vi "Z-Scan-test-1.vi"() -> ()   [LabVIEW 2014]
doc: "André Romero - 2016\nandretec@ifsc.usp.br"
uses:
  <vilib>/Utility/file.llb/Write To Spreadsheet File (DBL).vi
  <vilib>/Analysis/NI_AALBase.lvlib
panel:
  out "Waveform Chart 2":u32(graph)
  out "x-y":u32
  out "mean 2":dbl format="%0.2f"
  out "Waveform Chart":u32(graph)
  out "tempo":u32
  out "points":i32=1
  out "appended array":dbl[](array[numeric])
  out "variance":dbl format="%0.4f"
  out "standard deviation":dbl format="%0.4f"
  out "mean":dbl format="%0.4f"
  in  "Save ?":bool
  in  "delay between points (ms)":u32=100
  out "Waveform Graph 2":dbl[](graph)=[0.9929619826026088, 0.9923746873025917, 0.9818508984469507, 0.983827466273251, 0.9990107623733235, 1.0395239819940292, 0.9706500523861651, 1.06794722078419, 0.986424747001235, 1.0112744316316724, 0.9942522731444444, 1.001838469740766, 1.0029946225195683, 1.0126120902171765, 1.0021644811870658, 1.0061116820401748, 0.9972105448102168, 1.0068911643301743, 1.0052132138264187, 0.9992750904172452, 1.048311614015414, 0.9926080305613119, 1.0111948048086972, 0.9905398114026907, 1.0116783915731316, 0.98387502636871, 1.0107154218811778, 0.9941931066061604, 0.9875775120102475, 0.9829757035289887, 1.0188092280445085, 1.0111453402362722, 0.9875075292482545, 0.995337740298579, 1.0079138648082209, 1.0254835549800694, 0.9939970887218519, 0.9842725457434127, 0.9855748100955501, 0.9966738309822512, 1.0098279420600873, 0.9948048737150966, 1.0135979927834378, 0.964293348097744, 1.0004442713410568, 1.0081850647456483, 1.0302507900473072, 1.0228923303488178, 0.9667484984963655, 0.9865714477739775, 1.0364133365991077, 0.9977213956061421, 0.9832428050829438, 1.0383334543535299, 1.0096732459951854, 0.9825962938516749, 1.0183344805260317, 1.0177353873122412, 1.0225410223146796, 0.9860754307269641, 1.030312013840959, 1.0285466334678401, 1.0597004685457643, 0.9964393152435648, 1.0127420032997732, 1.0111564309410899, 0.9911153373064908, 0.9829525872811106, 0.9871642314547671, 1.0194200583287394, 1.00388773598447, 0.9746341672739159, 0.9904278906168584, 1.0033900330518635, 0.9936252883479672, 0.9845205151436855, 0.9945678585238711, 1.0016647654820403, 0.9879898688451537, 0.9863984551003344, 1.0110167839368691, 0.9752355124150663, 1.0344780794239226, 1.0122843072036265, 1.01049678196296, 0.970736922329293, 1.0241881965977657, 1.0115188722181554, 1.0293585291923657, 0.9982310438764077, 1.0051149836556408, 1.017911251728115, 0.9594139388753959, 1.0078413224573917, 1.003688804255993, 1.006221484876327, 0.9967339615841198, 1.0042760036472898, 0.9537852705680492, 1.0212543549523825, 1.0183418109287485, 0.9834384603549127, 0.9725833860677029, 0.9993225762516945, 1.002606361854476, 0.9876410897688062, 1.0036466615678723, 1.0019409165776714, 0.9963709181949384, 0.9968424660158376, 0.9935766114990483, 1.0116577111029135, 0.9882456586285582, 1.0072538601971548, 1.0120599790471025, 0.9770225341272584, 1.0173265485746734, 0.9723656657261552, 1.0043411013798933, 0.972400846287812, 0.9965743699288137, 1.0115957985488486, 1.0092600598782004, 1.028617902659787, 0.9756263120391087, 1.0251995340244466, 0.9981801685348355, 1.0172999638370765, 1.0056541703390969, 0.995990126879641, 0.9963655622831015, 1.032430445611457, 1.001431336754485, 1.0006099730723665, 1.0041724165772414, 1.0053778599068968, 0.991135402560612, 0.9998817432648112, 0.9912809462492138, 1.0035465593288295, 0.9882437595283899, 0.9782107765089285, 1.0228518124206731, 1.0087558934341563, 1.0241891638206257, 1.0193787553010976, 0.9921167807164234, 0.9927502420161048, 1.0107346398658508, 1.0188837238645847, 1.0221594671883125, 0.9965942993860635, 0.9842932321001923, 0.981847030230603, 0.9936136652990707, 0.9870447044168618, 0.9978949690731117, 0.9869918626920519, 0.9797386003847882, 1.0008386985082103, 1.0330280927007673, 1.004241674125628, 0.9909683650164001, 1.02695629802514, 1.0033708015406961, 1.0108056398846754, 0.9945908054831527, 1.0155686303054825, 0.985836754279153, 1.0122873083447073, 0.9813554692374822, 1.0073229755773239, 1.0020783249839669, 1.0023809695174208, 1.0021245575406161, 1.0074700445823073, 0.9899219659902431, 0.9881872351711627, 1.0049950341400478, 1.0046843040273437, 1.0201054172795425, 0.9937380855148645, 1.0021211500967366, 1.0088570028712045, 1.0044231329331996, 0.9984501684286005, 1.0013270763238702, 0.9774971335854716, 0.9866658163334106, 1.000980775430664, 0.9908481010755628, 1.0002528700293596, 0.9857656778619052, 0.9997826772620825, 1.0343649620339501, 1.0073234584006823, 0.9805240664825804, 1.0029654601008016, 0.9686768780166081, 1.0160258125494137, 1.0082079553664105, 0.9901357158841061, 0.994748065638555, 1.0052403943152382, 0.9871031757851597, 1.0214066887952424, 0.9704901116769896, 0.9950660968868316, 1.0019640529928464, 0.9936374248988875, 1.003497863963157, 1.0093061063561608, 0.9911483093985394, 0.997450965146168, 0.9966121176455948, 0.9993526179830612, 1.0053031425218377, 0.9913746748359868, 1.0026744008784367, 1.0025305796566382, 0.9931120665299722, 0.9864936832201258, 0.9828125296228193, 1.0154017305245813, 0.999977292098376, 1.003396060860759, 1.0090206669165798, 1.0124763635969498, 1.0105591289236533, 1.0084645494960998, 0.9855441101537715, 1.0017739263357615, 1.0065720022143287, 0.9922343777252469, 0.9981592542558017, 1.0001288888719242, 1.0039210730337789, 1.012377141773532, 1.0047424479160145, 1.0014599375745836, 1.013669723894066, 1.0050191875283112, 0.9938872072614322, 1.011570859686594, 0.996138314975225, 0.9939848274478382, 1.0065053877719619, 0.9944330961628688, 0.9791961444806913, 0.9999374454812969, 0.9975934276752868, 0.9944102204807054, 0.989392831994615, 1.0115392036215836, 1.0031898996148303, 1.0146271680824552, 0.9943257833943299, 0.9988752320358599, 1.0058922758561464, 1.006497779872354, 0.9930252211908878, 1.0235100479739772, 0.9933965078745319, 0.995734537346277, 0.9921857029695909, 0.997394921680454, 1.00664676734835, 1.0018598311217508, 0.999330072011583, 0.9988076745749431, 1.0106882210145283, 0.9964673682162559, 0.9977625424375128, 0.9969296445631848, 1.0097354699541692, 0.9908315377852488, 1.001406845754614, 0.9957275654561938, 0.9999071939760551, 1.0133978457034993, 1.0005501801740915, 0.9728144753536448, 0.9788149064050354, 0.9963338202361954, 0.9901746458167859, 1.0148500134459466, 1.0007813474773088, 1.0001239602007925, 1.0003956980130249, 0.9897066956415941, 1.0152655774500954, 1.006420164781569, 0.9987813936052027, 0.997929586836126, 1.0047079456911374, 0.9987477059026443, 0.9930327363838042, 0.997335295316322, 1.0006172967849036, 0.9833077793511378, 1.0085601133813822, 0.9943971410893149, 0.994239981170442, 1.0012084094477036, 0.9970289367786878, 0.9917988514890875, 1.000045439682172, 1.0047485655661257, 1.0030878243674637, 1.0023693825498734, 0.9823961549994707, 1.0089568692112538, 1.0128225400030877, 0.993059303619402, 1.0000477118317317, 1.008386816093551, 1.0061752524742424, 1.0012782594079208, 1.0088193880168852, 0.9998113759745942, 0.9916808751924095, 0.9947764469785467, 1.0000147588767094, 1.004168257302679, 1.0049594024199107, 0.9976032955590068, 0.9950024479190206, 1.0010719492755789, 0.996495733920656, 0.9931299914854711, 0.9996314626869472, 0.9967261318393039, 1.0017881000228432, 0.9996299959948114, 1.0101811967459287, 0.9972172980755194, 1.0026876373677753, 1.0086980306140763, 0.9945815124225268, 0.992232697319385, 0.9959716654440998, 0.9837072672693644, 0.998613413654516, 1.0033460606080056, 0.9922003296634196, 0.9970686937119227, 0.9947857405409758, 1.0033550767809771, 1.009532678928252, 1.004991391987436, 1.0012506544173572, 0.9992373958872778, 0.9896683840618742, 1.0111383485139052, 0.9997228671391453, 0.9959069824783411, 0.9956385118276566, 1.0000596218314721, 1.0022790874156704, 0.9934387624412249, 1.0120554243504905, 1.0082592470120304, 0.9912363155165209, 1.0083861710662205, 1.0003750950383337, 0.991199648091011, 0.9949674643665423, 0.9997959886665277, 1.0030465165685307, 1.017871899016287, 1.0021625648413868, 1.001580064304153, 0.9997002178450737, 1.002128209587292, 1.0060096072639728, 0.996254399347374, 1.0024668985501985, 0.9980621968183131, 1.0050577276864496, 1.007087038917439, 1.0106503628134398, 1.0067084285722847, 1.013698164804235, 0.9925226618865702, 1.003698876241974, 1.002416705988079, 1.0042322322725372, 1.0002681428339832, 0.9874053999281158, 0.9949182725925264, 0.9886789045049351, 0.9867770197005105, 0.995571098062274, 0.9943171527111376, 0.9924453729346618, 1.011359442849128, 1.000050925690945, 1.0038097355051494, 1.0040083211266855, 0.9959692610441326]
  in  "N Points":i32=100
  in  "stop":bool
  out "graph":dbl[][](graph)
  in  "N samples":i32=8000
  in  "rate":dbl=50000.0
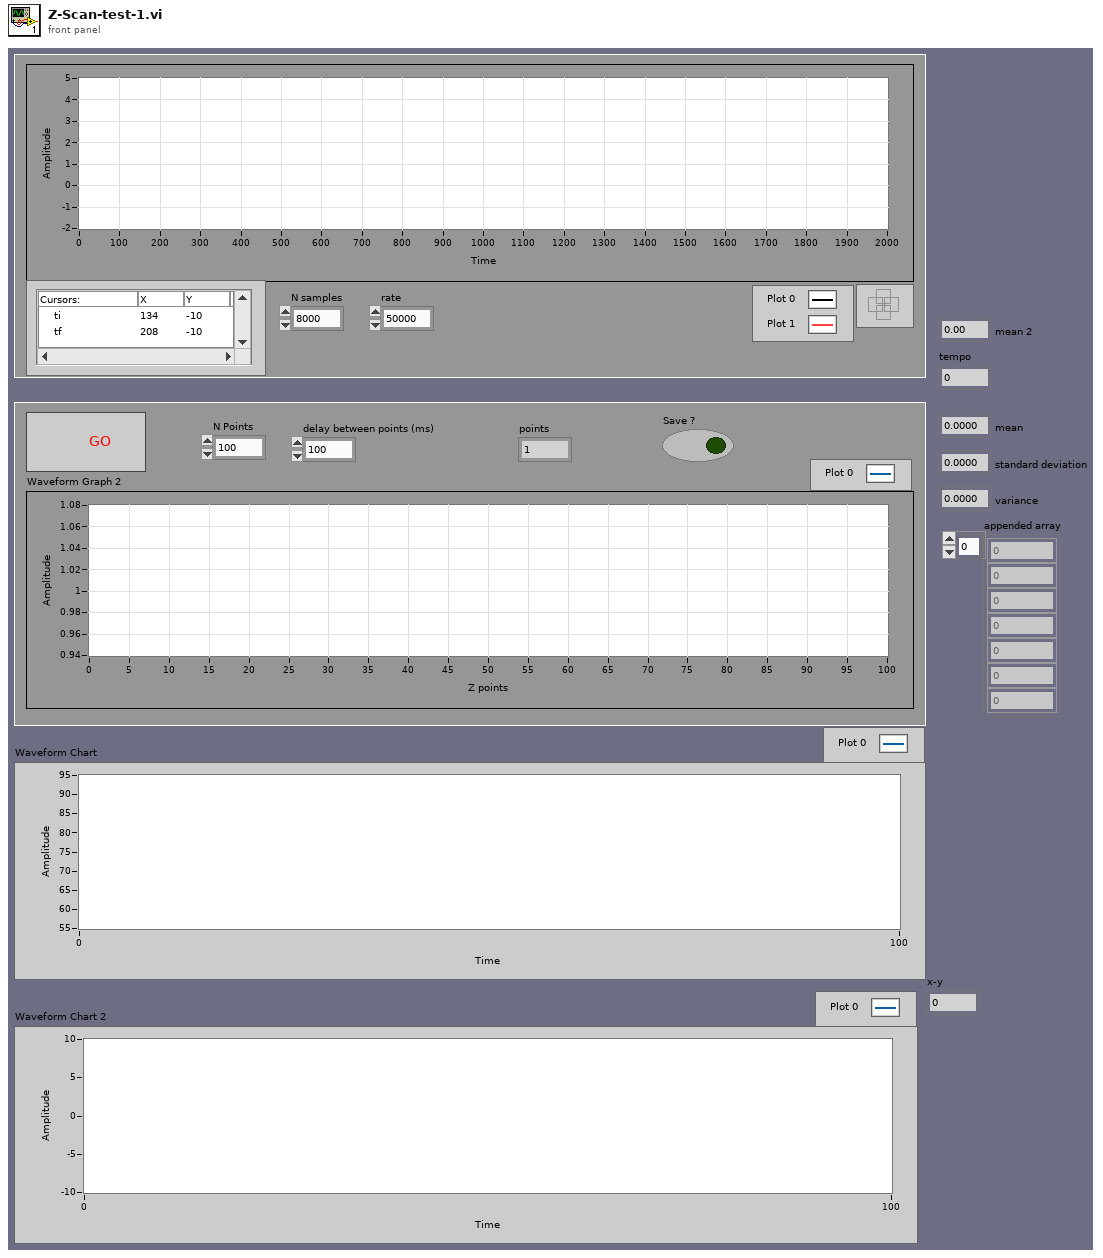
[diagram p1: front panel]
types:
  T1 = typedef "LVCursorListTypeDef.ctl" = cluster{"Name":string, "Color":u32, "Style":u8, "Point Style":u8, "Name Visible":bool, "Allow Drag":bool, "Cursor Mode":u32, "Plot":i32, "Index":i32, "Position":cluster{"X":dbl, "Y":dbl}, "X Scale":u32, "Y Scale":u32, "Watch Plots":i32[], "Watch All Plots":bool, "Plot Area":i32, "Label Offset":cluster{"X":dbl, "Y":dbl}}[]
  T2 = cluster{"Name":string, "Color":u32, "Style":u8, "Point Style":u8, "Name Visible":bool, "Allow Drag":bool, "Cursor Mode":u32, "Plot":i32, "Index":i32, "Position":cluster{"X":dbl, "Y":dbl}, "X Scale":u32, "Y Scale":u32, "Watch Plots":i32[], "Watch All Plots":bool, "Plot Area":i32, "Label Offset":cluster{"X":dbl, "Y":dbl}}
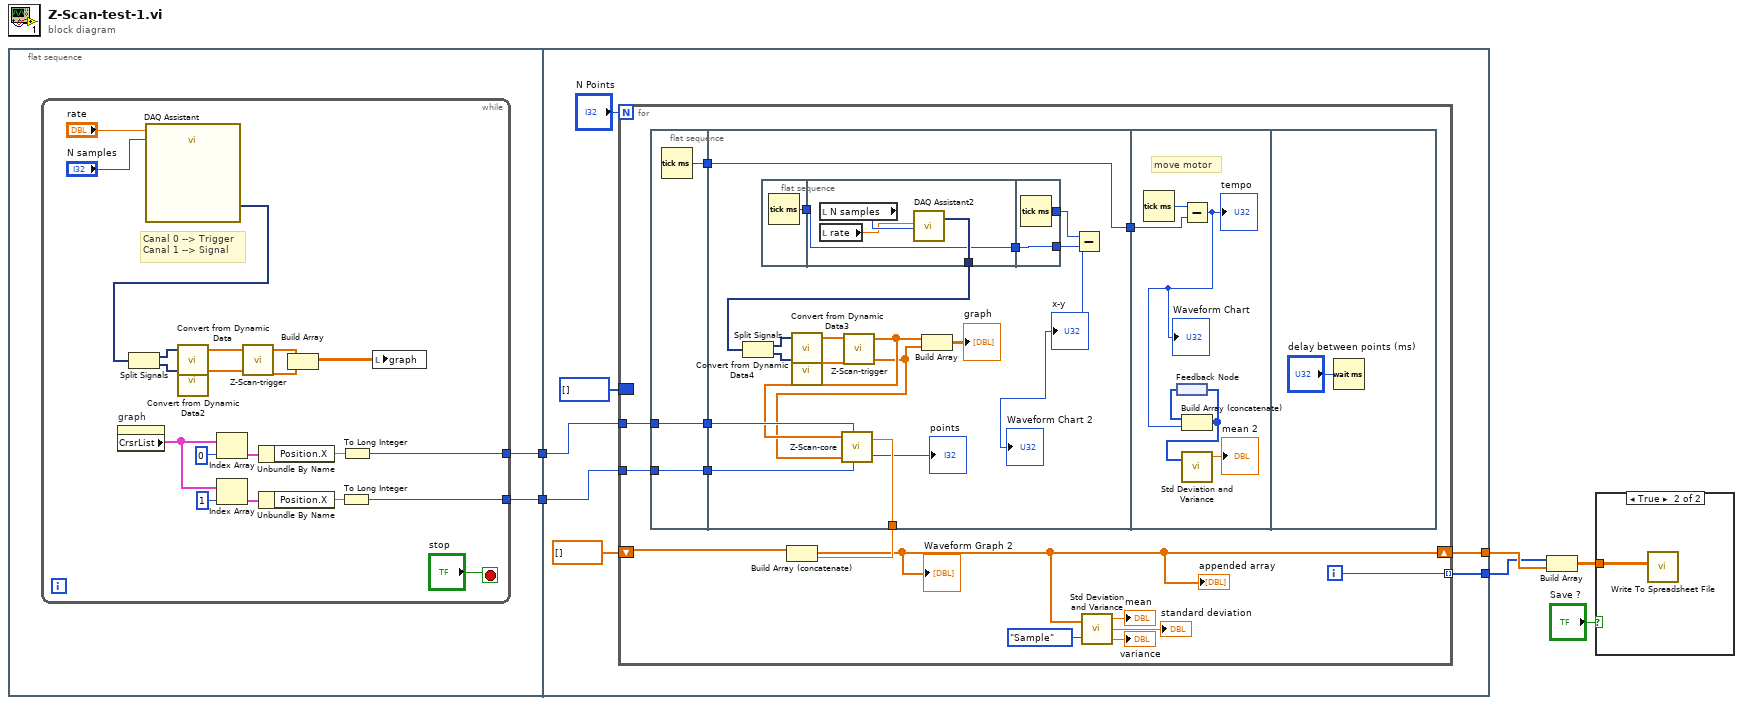
[diagram p0: block diagram]
diagram:
  n1 = flat-sequence {
    tunnel: [w8] -> w6
    tunnel: [w7] -> w5
    tunnel: w6 -> [w34]
    tunnel: w5 -> [w33]
    tunnel: [w32] -> w4
    tunnel: [w31] -> w3
    frame #0 {
      n2 = while {
        tunnel: [w16] -> w8
        tunnel: [w15] -> w7
        stop <- "stop" stop-if-true
        # "Canal 0 --> Trigger\nCanal 1 --> Signal"
        n3 = property on="graph" class="WFGraph (strict)"() -> ("CrsrList"=w22:T1)  [unwired: 2 in, 2 out]
        n4 = call "DAQ Assistant"("rate"="rate", "number of samples"="N samples") -> ("data"=w24:dynamicdata)  [unwired: 15 in, 2 out]
        n5 = Split Signals(w24) -> (w26:dynamicdata, w25:dynamicdata)  [unwired: 2 in]
        n6 = call "Convert from Dynamic Data"("Dynamic Data Type"=w26) -> ("Array"=w12:dbl[])  [unwired: 3 in]
        n7 = call "Convert from Dynamic Data2"("Dynamic Data Type"=w25) -> ("Array"=w11:dbl[])  [unwired: 3 in]
        n8 = Index Array(array=w22, index=0) -> (element=w20:T2)
        n9 = Index Array(array=w22, index=1) -> (element=w19:T2)
        n10 = call "Z-Scan-trigger.vi"("trigger in"=w12, "signal in"=w11) -> ("trigger out"=w14:dbl[], "signal out"=w9:dbl[])  [unwired: 4 in]
        n11 = Unbundle By Name(w20) -> ("Position.X"=w18:dbl)
        n12 = Unbundle By Name(w19) -> ("Position.X"=w17:dbl)
        n13 = Build Array(w9, w14) -> (w10:dbl[][])
        n14 = To Long Integer(number=w17) -> (32bit integer=w15:i32)
        n15 = To Long Integer(number=w18) -> (32bit integer=w16:i32)
        n16 = local write "graph"(w10) -> ()
      }
    }
    frame #1 {
      n17 = for {
        N: "N Points" -> [_]
        tunnel: w34 -> [w49]
        tunnel: w33 -> [w48]
        shift-right: [w41] -> w32
        shift-left: dbl[] [] -> [w47]
        tunnel: [w45] -> w31 mode=indexing
        border: u32[] [] -> [_]
        i -> [w45]
        n18 = flat-sequence {
          tunnel: w48 -> [w51]
          tunnel: w49 -> [w52]
          tunnel: [w52] -> w39
          tunnel: [w51] -> w38
          tunnel: [w50] -> w36
          tunnel: [w64] -> w46
          tunnel: w39 -> [w66]
          tunnel: w38 -> [w65]
          tunnel: [w59] -> w37
          tunnel: w36 -> [w59]
          tunnel: w37 -> [w82]
          frame #0 {
            n19 = Tick Count (ms)() -> (millisecond timer value=w50:u32)
          }
          frame #1 {
            n20 = Split Signals(w58) -> (w70:dynamicdata, w69:dynamicdata)  [unwired: 2 in]
            n21 = flat-sequence {
              tunnel: [w71] -> w54
              tunnel: [w73] -> w58
              tunnel: [w72] -> w55
              tunnel: w54 -> [w72]
              tunnel: [w77] -> w57
              tunnel: [w76] -> w56
              tunnel: w55 -> [w76]
              frame #0 {
                n22 = Tick Count (ms)() -> (millisecond timer value=w71:u32)
              }
              frame #1 {
                n23 = local read "N samples"() -> (w75:i32)
                n24 = local read "rate"() -> (w74:dbl)
                n25 = call "DAQ Assistant2"("rate"=w74, "number of samples"=w75) -> ("data"=w73:dynamicdata)  [unwired: 15 in, 2 out]
              }
              frame #2 {
                n26 = Tick Count (ms)() -> (millisecond timer value=w77:u32)
              }
            }
            n27 = call "Convert from Dynamic Data3"("Dynamic Data Type"=w70) -> ("Array"=w68:dbl[])  [unwired: 3 in]
            n28 = call "Convert from Dynamic Data4"("Dynamic Data Type"=w69) -> ("Array"=w67:dbl[])  [unwired: 3 in]
            n29 = call "Z-Scan-trigger.vi"("trigger in"=w68, "signal in"=w67) -> ("trigger out"=w63:dbl[], "signal out"=w61:dbl[])  [unwired: 4 in]
            n30 = call "Z-Scan-core.vi"("trigger in"=w63, "ti"=w66, "signal in"=w61, "tf"=w65) -> ("mean tf/ti"=w64:dbl, "number of samples"=→"points":i32)  [unwired: 1 in]
            n31 = Build Array(w63, w61) -> (→"graph":dbl[][])
            n32 = Subtract(x=w57, y=w56) -> (x-y=→"x-y" →"Waveform Chart 2":u32)
          }
          frame #2 {
            # "move motor"
            n33 = Tick Count (ms)() -> (millisecond timer value=w83:u32)
            n34 = feedback #1() -> (w81:u32[])
            n35 = Subtract(x=w83, y=w82) -> (x-y=w80:u32)
            "tempo" <- w80
            "Waveform Chart" <- w80
            n36 = Build Array (concatenate)(w81, w80) -> (w79:u32[])
            n37 = feedback-in #1(w79) -> ()
            n38 = call <vilib>:"Std Deviation and Variance.vi"("X"=w79) -> ("mean"=→"mean 2":dbl)  [unwired: 1 in, 2 out]
          }
          frame #3 {
            n39 = Wait (ms)(milliseconds to wait="delay between points (ms)") -> ()  [unwired: 1 out]
          }
        }
        n40 = Build Array (concatenate)(w47, w46) -> (w41:dbl[])
        "Waveform Graph 2" <- w41
        "appended array" <- w41
        n41 = call <vilib>:"Std Deviation and Variance.vi"("X"=w41, "Weighting (Sample)"=enum16{"Sample", "Population"}."Sample") -> ("mean"=→"mean":dbl, "standard deviation"=→"standard deviation":dbl, "variance"=→"variance":dbl)
      }
    }
  }
  n42 = Build Array(w3, w4) -> (w1:dbl[][])
  n43 = case shown="True" "Save ?" {
    tunnel: w1 -> [_ w85]
    frame False {
    }
    frame True {
      n44 = call-poly <vilib>:"Write To Spreadsheet File.vi"("2D data"=w85) -> ()  [unwired: 7 in, 1 out]
    }
  }
